vi "Recieve Request for Result.vi"(6 "Request time":timestamp, 8 "error in (no error)":errorcluster, 9 "Requestor":string, 10 "Requestee":string, 11 "Red Pitaya in":refnum<class "Red Pitaya.lvclass">) -> (0 "error out":errorcluster, 3 "Red Pitaya out":refnum<class "Red Pitaya.lvclass">)   [LabVIEW 2015, in "Red Pitaya.lvclass"]
uses:
  Red Pitaya.lvclass
  Red Pitaya.lvclass/Red Pitaya.ctl
  Mag Lab Measure/Hardware/Spectrum Analyzer/Spectrum Analyzer.lvclass/Spectrum Analyzer.ctl
  Mag Lab Measure/Mag Lab Root Messages/Recieve Request for Result Msg/Recieve Request for Result Msg.lvclass
  Mag Lab Measure/Mag Lab Root Messages/Recieve Request for Result Msg/Recieve Request for Result Msg.lvclass/Recieve Request for Result Msg.ctl
  <vilib>/ActorFramework/Actor/Actor.lvclass/Actor.ctl
  Mag Lab Measure/Mag Lab Result/Scaled I32 Array Result/Scaled I32 Array Result.lvclass
  Mag Lab Measure/Mag Lab Result/Mag Lab Result.lvclass/Mag Lab Result.ctl
  Mag Lab Measure/Mag Lab Result/Scaled I32 Array Result/Scaled I32 Array Result.lvclass/Scaled I32 Array Result.ctl
  Mag Lab Measure/Mag Lab Root Messages/Recieve Response with Result Msg/Recieve Response with Result Msg.lvclass/Recieve Response with Result Msg.ctl
  <vilib>/ActorFramework/Message Enqueuer/Message Enqueuer.lvclass/Message Enqueuer.ctl
  Mag Lab Measure/Hardware/Spectrum Analyzer/Read Frequencies.vi
  Mag Lab Measure/Mag Lab Root Messages/Recieve Request for Result Msg/Write Requestee.vi
  Mag Lab Measure/Mag Lab Root Messages/Recieve Request for Result Msg/Write Requestor.vi
  Mag Lab Measure/Mag Lab Root Messages/Recieve Request for Result Msg/Write Request time.vi
  Mag Lab Measure/Mag Lab Result/Write Group Name.vi
  Mag Lab Measure/Mag Lab Result/Write Name.vi
  Mag Lab Measure/Mag Lab Result/Scaled I32 Array Result/Write Channel names.vi
  Mag Lab Measure/Mag Lab Result/Scaled I32 Array Result/Write I32 Array.vi
  Mag Lab Measure/Mag Lab Result/Scaled I32 Array Result/Write Scale Array.vi
  Mag Lab Measure/Mag Lab Result/Write Result time.vi
  <vilib>/ActorFramework/Message Enqueuer/Enqueue.vi
  <vilib>/ActorFramework/Message Priority Queue/Priority Enqueue.vi
  Mag Lab Measure/Mag Lab Root Messages/Recieve Response with Result Msg/Recieve Response with Result Msg.lvclass
  <vilib>/ActorFramework/Actor/Actor.lvclass
  Mag Lab Measure/Mag Lab Error Handler/Mag Lab Error Handler.lvclass
  Mag Lab Measure/Hardware/Spectrum Analyzer/Spectrum Analyzer.lvclass
panel:
  out "Output Fifo cnt":i32
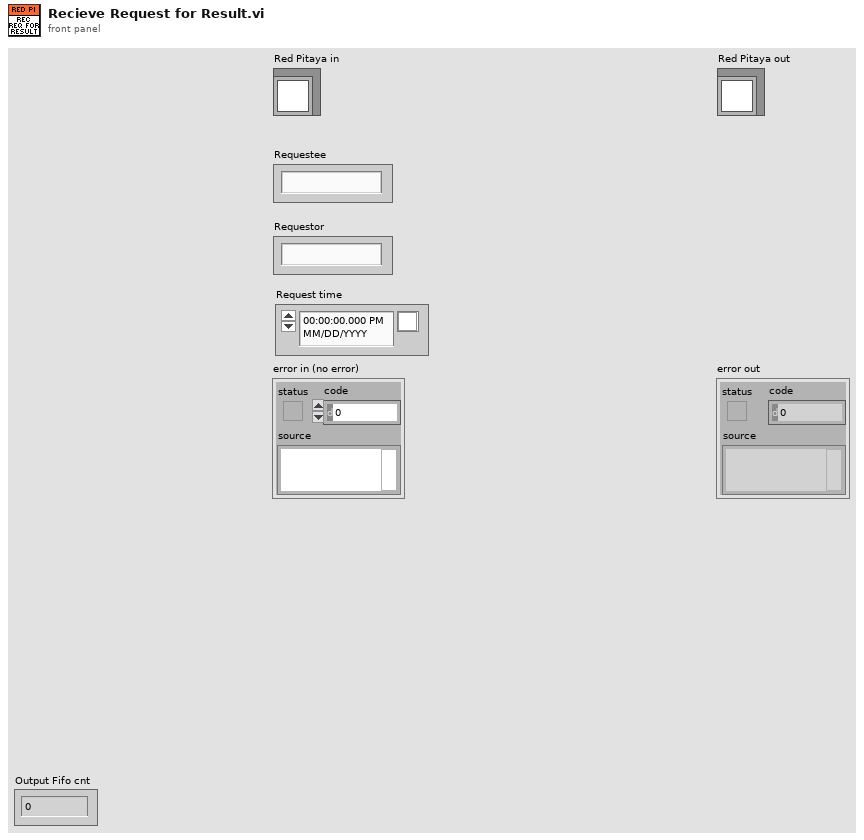
[diagram p1: front panel]
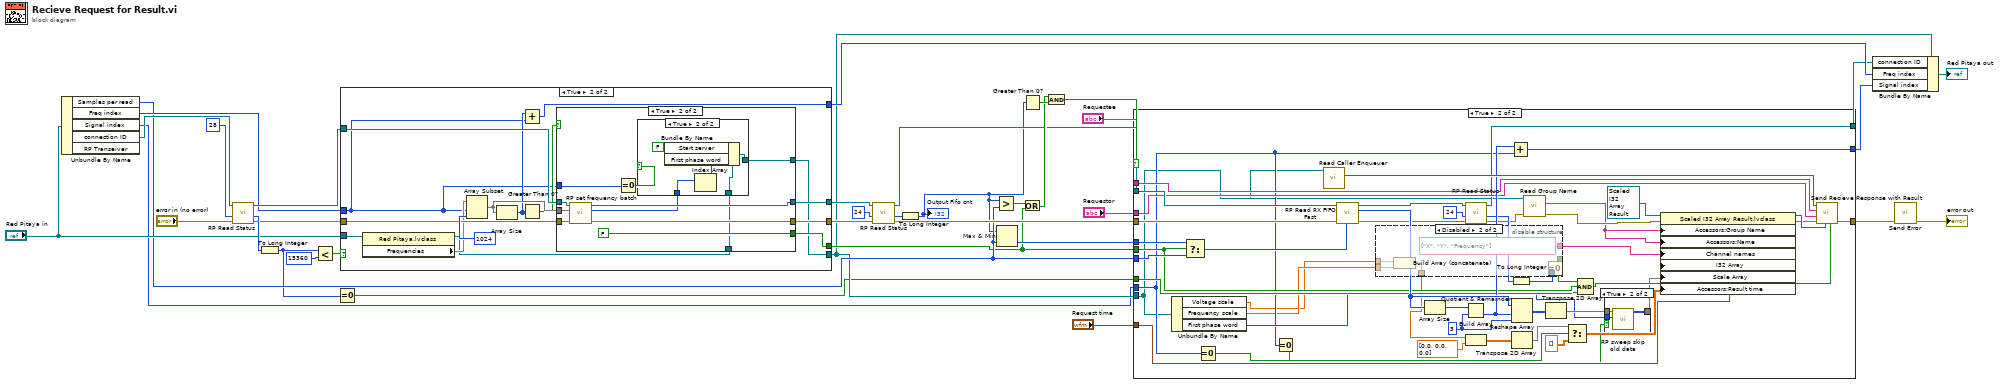
[diagram p0: block diagram]
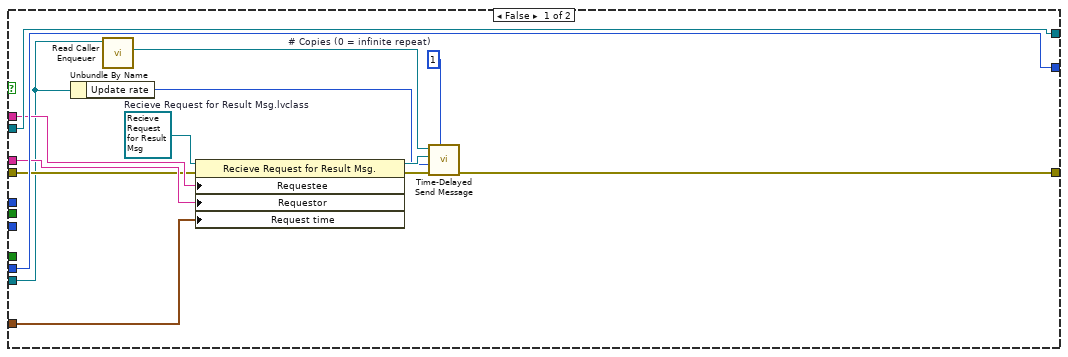
[diagram p2: hidden frame]
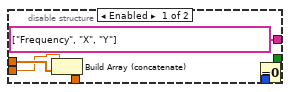
[diagram p3: hidden frame]
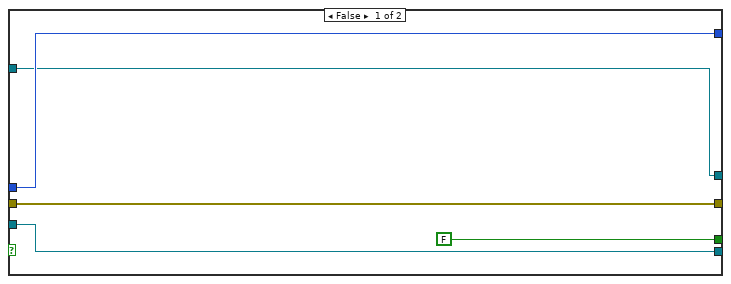
[diagram p5: hidden frame]
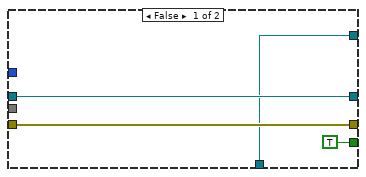
[diagram p6: hidden frame]
diagram:
  n1 = Unbundle By Name("Red Pitaya in") -> ("Samples per read"=w15:i32, "Freq index"=w30:i32, "Signal index"=w9:i32, "connection ID"=w35:refnum<k5>)  [unwired: 1 out]
  n2 = call "RP Read Status.vi"("Error In"="error in (no error)", "Status offset"=u64 28, "connection ID"=w35) -> ("Error Out"=w32:errorcluster, "Status response"=w36:u32, "connection ID out"=w31:refnum<k5>)  [unwired: 6 in]
  n3 = To Long Integer(number=w36) -> (32bit integer=w13:i32)
  n4 = Less?(x=w13, y=15360) -> (x < y?=w28:bool)
  n5 = Equal To 0?(x=w13) -> (x = 0?=w1:bool)
  n6 = case shown="True" w28 {
    tunnel: w30 -> [w42 w45]
    tunnel: [w42 w56] -> w29
    tunnel: w32 -> [w40 w55]
    tunnel: w31 -> [w41 w54]
    tunnel: [w41 w53] -> w16
    tunnel: [w40 w52] -> w17
    tunnel: [FALSE w49] -> w12
    tunnel: "Red Pitaya in" -> [w39 w47]
    tunnel: [w39 w43] -> w11
    frame False {
    }
    frame True {
      n7 = property class="Red Pitaya.lvclass"(reference=w47) -> (reference out=w44:refnum<class "Red Pitaya.lvclass">, "Frequencies"=w46:dbl[])  [unwired: 1 in, 1 out]
      n8 = Array Subset(array=w46, index=w45, length=1024) -> (w51:dbl[])
      n9 = Array Size(array=w51) -> (size(s)=w48:i32)
      n10 = Add(x=w48, y=w45) -> (x+y=w56:i32)
      n11 = Greater Than 0?(x=w48) -> (x > 0?=w50:bool)
      n12 = case shown="True" w50 {
        tunnel: w55 -> [w61 w72]
        tunnel: w54 -> [w60 w71]
        tunnel: [w60 w70] -> w53
        tunnel: [w61 w69] -> w52
        tunnel: w51 -> [_ w68]
        tunnel: [TRUE FALSE] -> w49
        tunnel: w45 -> [_ w66]
        tunnel: w44 -> [w58 w63]
        tunnel: [w58 w62] -> w43
        frame False {
        }
        frame True {
          n13 = call "RP set frequency batch.vi"("Error In"=w72, "Frequency"=w68, "connection ID"=w71) -> ("Error Out"=w69:errorcluster, "Phase words sent"=w64:u32[], "connection ID out"=w70:refnum<k5>)  [unwired: 6 in]
          n14 = Equal To 0?(x=w66) -> (x = 0?=w65:bool)
          n15 = case shown="True" w65 {
            tunnel: w64 -> [_ w78]
            tunnel: w63 -> [w73 w77]
            tunnel: [w73 w75] -> w62
            frame False {
            }
            frame True {
              n16 = Index Array(array=w78) -> (element=w76:u32)  [unwired: 1 in]
              n17 = Bundle By Name(cluster=w77, "Start server"=FALSE ("Found first"), "First phase word"=w76) -> (w75:refnum<class "Red Pitaya.lvclass">)
            }
          }
        }
      }
    }
  }
  n18 = call "RP Read Status.vi"("Error In"=w17, "Status offset"=u64 24, "connection ID"=w16) -> ("Error Out"=w21:errorcluster, "Status response"=w19:u32, "connection ID out"=w20:refnum<k5>)  [unwired: 6 in]
  n19 = To Long Integer(number=w19) -> (32bit integer=w14:i32)
  "Output Fifo cnt" <- w14
  n20 = Greater?(x=w14, y=w15) -> (0:w23:bool)
  n21 = Max & Min(x=w14, y=w15) -> (min(x,y)=w26:i32)  [unwired: 1 out]
  n22 = Greater Than 0?(x=w14) -> (x > 0?=w25:bool)
  n23 = Or(x=w23, y=w12) -> (x .or. y?=w22:bool)
  n24 = And(x=w22, y=w25) -> (x .and. y?=w24:bool)
  n25 = case shown="True" w24 {
    tunnel: w20 -> [w92 w141]
    tunnel: w21 -> [w86 w140]
    tunnel: [w82 w120] -> w6
    tunnel: [w92 w113] -> w7
    tunnel: w15 -> [_ w137]
    tunnel: w26 -> [_ w138]
    tunnel: w12 -> [_ w112]
    tunnel: w11 -> [w81 w100]
    tunnel: w9 -> [w91 w102]
    tunnel: [w91 w127] -> w8
    tunnel: "Request time" -> [w87 w119]
    tunnel: "Requestee" -> [w89 w118]
    tunnel: "Requestor" -> [w88 w117]
    tunnel: w1 -> [_ w107]
    frame False {
      w79 = u32 1  # # Copies (0 = infinite repeat)
      w90 = refnum<class "Recieve Request for Result Msg.lvclass"> refnum  # Recieve Request for Result Msg.lvclass
      n26 = Unbundle By Name(w81) -> ("Update rate"=w80:i32)
      n27 = call <vilib>:"Read Caller Enqueuer.vi"("Actor"=w81) -> ("Caller Enqueuer"=w83:refnum<class "Message Enqueuer.lvclass">)  [unwired: 10 in]
      n28 = property class="Recieve Request for Result Msg."(reference=w90, error in=w86, "Requestee"=w89, "Requestor"=w88, "Request time"=w87) -> (reference out=w85:refnum<class "Recieve Request for Result Msg.lvclass">, error out=w84:errorcluster)
      n29 = call <vilib>:"Time-Delayed Send Message.vi"("# Copies (0 = infinite repeat)"=w79, "error in (no error)"=w84, "Milliseconds To Wait"=w80, "Message"=w85, "Message Enqueuer"=w83) -> ("error out"=w82:errorcluster)  [unwired: 5 in, 1 out]
    }
    frame True {
      w129 = 3 ("dimension size")
      n30 = Unbundle By Name(w100) -> ("Voltage scale"=w94:dbl[], "Frequency scale"=w95:dbl, "First phase word"=w103:u32)
      n31 = Select(t=w138, s=w112, f=w137) -> (s? t:f=w139:i32)
      n32 = Equal To 0?(x=w102) -> (x = 0?=w126:bool)
      n33 = Equal To 0?(x=w102) -> (x = 0?=w101:bool)
      n34 = call "RP Read RX FIFO Fast.vi"("Samples per read"=w139, "Error In"=w140, "connection ID"=w141) -> ("Error Out"=w115:errorcluster, "FIFO out"=w130:i32[], "connection ID out"=w114:refnum<k5>)  [unwired: 6 in]
      n35 = Array Size(array=w130) -> (size(s)=w133:i32)
      n36 = call "RP Read Status.vi"("Error In"=w115, "Status offset"=u64 24, "connection ID"=w114) -> ("Error Out"=w98:errorcluster, "Status response"=w111:u32, "connection ID out"=w113:refnum<k5>)  [unwired: 6 in]
      n37 = Quotient & Remainder(x=w133, y=w129) -> (floor(x/y)=w128:i32)  [unwired: 1 out]
      n38 = Add(x=w128, y=w102) -> (x+y=w127:i32)
      n39 = To Long Integer(number=w111) -> (32bit integer=w110:i32)
      n40 = disable-structure shown="Disabled" {
        disable-tunnel: w110 -> [w147 w153]
        disable-tunnel: [w146 w152] -> w108
        disable-tunnel: [string[] ["Frequency", "X", "Y"] ("Channel names") string[] ["X", "Y", "Frequency"] ("Channel names")] -> w106
        disable-tunnel: w95 -> [w143 w149]
        disable-tunnel: w94 -> [w144 w150]
        disable-tunnel: [w142 w148] -> w93
        frame Enabled {
          n41 = Build Array (concatenate)(w143, w144) -> (w142:dbl[])
          n42 = Equal To 0?(x=w147) -> (x = 0?=w146:bool)
        }
        frame Disabled {
          n43 = Build Array (concatenate)(w150, w149) -> (w148:dbl[])
          n44 = Equal To 0?(x=w153) -> (x = 0?=w152:bool)
        }
      }
      n45 = Build Array(w93, dbl[] [0.0, 0.0, 0.0] ("element")) -> (w124:dbl[][])
      n46 = Reshape Array(w130, w128, w129) -> (w132:i32[][])
      n47 = Transpose 2D Array(2D array=w124) -> (transposed array=w123:dbl[][])
      n48 = call "Read Group Name.vi"("error in (no error)"=w98, "Spectrum Analyzer in"=w100) -> ("error out"=w97:errorcluster, "Group Name"=w96:string, "Spectrum Analyzer out"=w99:refnum<class "Red Pitaya.lvclass">)  [unwired: 7 in]
      n49 = call <vilib>:"Read Caller Enqueuer.vi"("Actor"=w99) -> ("Caller Enqueuer"=w135:refnum<class "Message Enqueuer.lvclass">)  [unwired: 10 in]
      n50 = Transpose 2D Array(2D array=w132) -> (transposed array=w131:i32[][])
      n51 = Select(t=w123, s=w126, f=dbl[][] []) -> (s? t:f=w121:dbl[][])
      n52 = Compound Arithmetic op=AND(w108, w112, w107) -> (w105:bool)
      n53 = case shown="True" w101 {
        tunnel: w131 -> [w154 w157]
        tunnel: [w154 w156] -> w104
        tunnel: w103 -> [_ w155]
        frame False {
        }
        frame True {
          n54 = call "RP sweep skip old data.vi"("First new data"=w155, "Input stream"=w157) -> ("Output stream"=w156:i32[][])  [unwired: 8 in, 1 out]
        }
      }
      n55 = property class="Scaled I32 Array Result.lvclass"(reference=refnum<class "Scaled I32 Array Result.lvclass"> refnum ("Scaled I32 Array Result.lvclass"), error in=w97, "Accessors:Group Name"=w96, "Accessors:Name"=w96, "Channel names"=w106, "I32 Array"=w104, "Scale Array"=w121, "Accessors:Result time"=w119) -> (reference out=w134:refnum<class "Scaled I32 Array Result.lvclass">, error out=w109:errorcluster)
      n56 = call "Send Recieve Response with Result.vi"("Finished"=w105, "Result"=w134, "error in (no error)"=w109, "Requestor"=w117, "Requestee"=w118, "Message Enqueuer"=w135) -> ("error out"=w120:errorcluster)  [unwired: 4 in, 1 out]
    }
  }
  n57 = Bundle By Name(cluster=w11, "connection ID"=w7, "Freq index"=w29, "Signal index"=w8) -> (→"Red Pitaya out":refnum<class "Red Pitaya.lvclass">)
  n58 = call "Send Error.vi"("error in (no error)"=w6) -> ("error out"=→"error out":errorcluster)  [unwired: 9 in, 1 out]
